vi "GCode_SetZero_G92.vi"(11 "?":cluster{"X":dbl, "Y":dbl, "Z":dbl}) -> (3 "String":string)   [LabVIEW 2017]
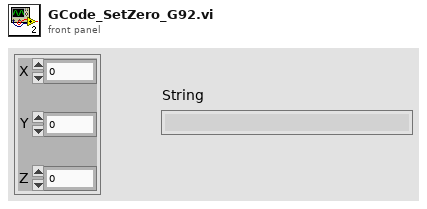
[diagram p1: front panel]
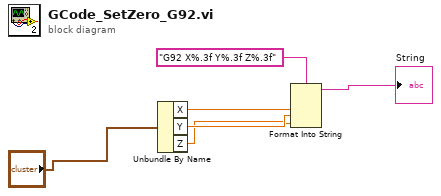
[diagram p0: block diagram]
diagram:
  n1 = Unbundle By Name("?") -> ("X"=w3:dbl, "Y"=w2:dbl, "Z"=w1:dbl)
  n2 = Format Into String(format string="G92 X%.3f Y%.3f Z%.3f", w3, w2, w1) -> (resulting string=→"String":string)  [unwired: 2 in, 1 out]
